vi "Get Tree Value.vi"(11 "UI Data in":refnum<class "Settings UI.lvclass">) -> (2 "Value":string, 3 "UI Data out":refnum<class "Settings UI.lvclass">)   [LabVIEW 2020, in "Output Sequencer.lvlib" / "Settings UI.lvclass"]
uses:
  Settings UI.lvclass
  Settings UI.lvclass/Settings UI.ctl
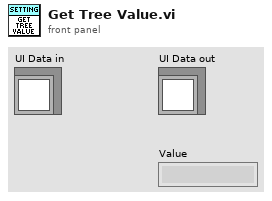
[diagram p1: front panel]
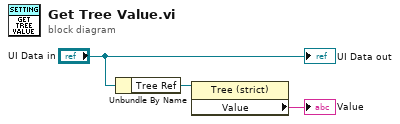
[diagram p0: block diagram]
diagram:
  n1 = Unbundle By Name("UI Data in") -> ("Tree Ref"=w1:refnum<vi>)
  n2 = property class="Tree (strict)"(reference=w1) -> ("Value"=→"Value":string)  [unwired: 1 in, 2 out]
  "UI Data out" <- "UI Data in"
